vi "Package Data.vi"(8 "error in (no error)":errorcluster, 10 "DataIn":string, 11 "M data in":refnum<class "M data.lvclass">) -> (0 "error out":errorcluster, 3 "M data out":refnum<class "M data.lvclass">)   [LabVIEW 2014, in "M data.lvclass"]
uses:
  M data.lvclass
  M data.lvclass/M data.ctl
  reusable/General/Atmospheric/Atmospheric Constants.vi
  reusable/Data/Write measTime.vi
  reusable/General/Atmospheric/Atmospheric Library.lvlib
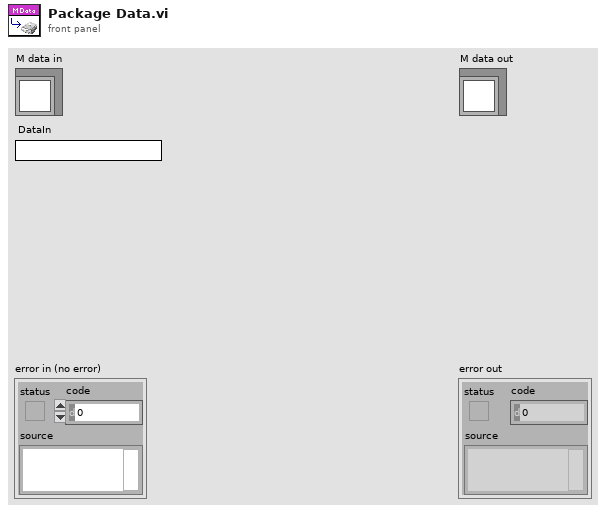
[diagram p1: front panel]
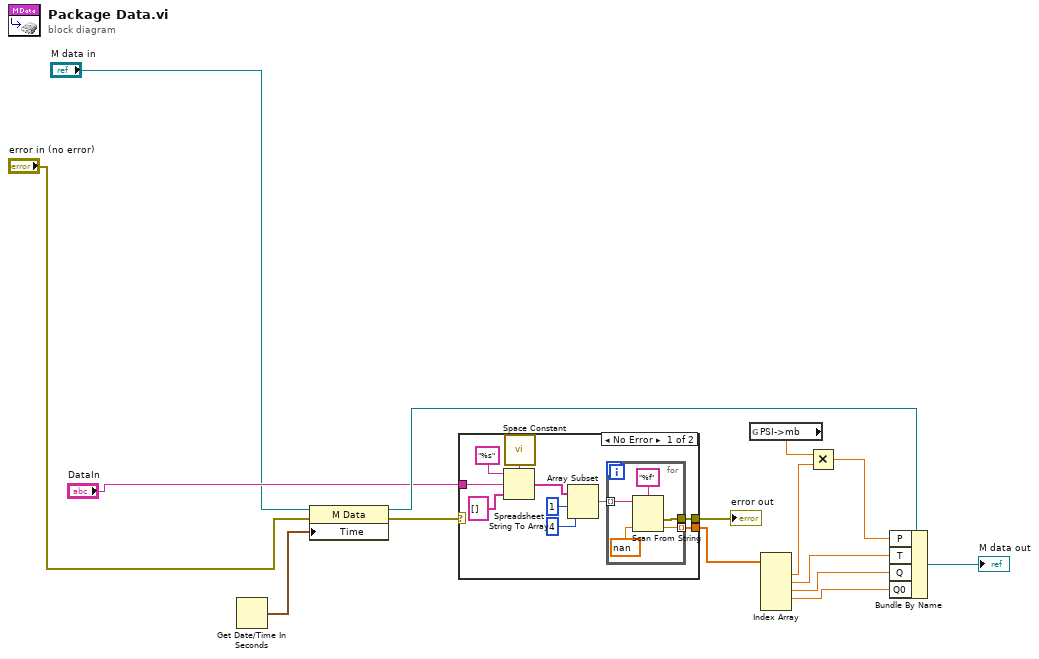
[diagram p0: block diagram]
diagram:
  n1 = Get Date/Time In Seconds() -> (seconds since 1Jan1904=w6:timestamp)
  n2 = property class="M Data"(reference="M data in", error in="error in (no error)", "Time"=w6) -> (reference out=w8:refnum<class "M data.lvclass">, error out=w7:errorcluster)
  n3 = case shown="No Error" w7 {
    selector: w7 -> [_ w31]
    tunnel: "DataIn" -> [w22 _]
    tunnel: [w17 _] -> w9
    tunnel: [w21 w31] -> w2
    frame No Error {
      n4 = call <vilib>:"Space Constant.vi"() -> ("String"=w24:string)
      n5 = Spreadsheet String To Array(delimiter (Tab)=w24, format string="%s", spreadsheet string=w22, array type (2D Dbl)=string[] []) -> (array=w20:string[])
      n6 = Array Subset(array=w20, index=1, length=4) -> (w18:string[])
      n7 = for {
        tunnel: w18 -> [w26] mode=indexing
        tunnel: [w28] -> w17 mode=indexing
        tunnel: [w27] -> w21
        n8 = Scan From String(format string="%f", input string=w26, default 1=sgl nan ("default value 1")) -> (error out=w27:errorcluster, output 1=w28:sgl)  [unwired: 2 in, 2 out]
      }
    }
    frame Error {
    }
  }
  "error out" <- w2
  n9 = global read "Atmospheric Constants.vi" "PSI->mb"() -> (w10:sgl)
  n10 = Index Array(array=w9) -> (element #1=w14:sgl, element #2=w13:sgl, element #3=w12:sgl, element #4=w11:sgl)  [unwired: 5 in, 1 out]
  n11 = Multiply(x=w10, y=w14) -> (x*y=w15:sgl)
  n12 = Bundle By Name(cluster=w8, "P"=w15, "T"=w13, "Q"=w12, "Q0"=w11) -> (→"M data out":refnum<class "M data.lvclass">)
